vi "Read command in.vi"(8 "error in (no error)":errorcluster, 11 "Motor in":refnum<class "Motor.lvclass">) -> (0 "error out":errorcluster, 1 "action not empty":bool, 2 "command in":T1, 3 "Motor out":refnum<class "Motor.lvclass">)   [LabVIEW 2018, in "Motor.lvclass"]
uses:
  Motor.lvclass
  Motor.lvclass/Motor.ctl
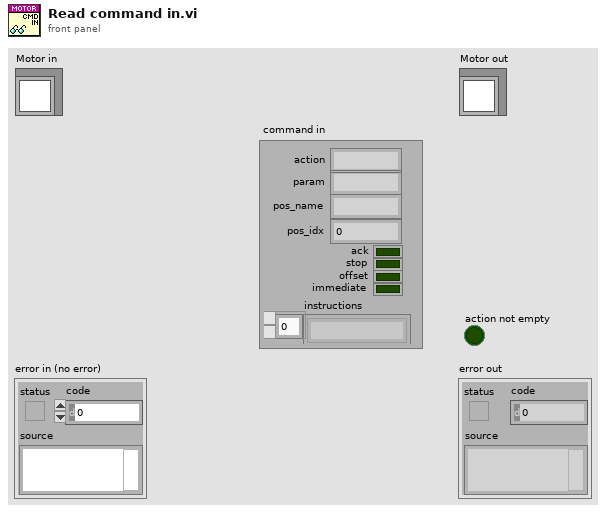
[diagram p1: front panel]
types:
  T1 = cluster{"action":string, "param":string, "pos_name":string, "pos_idx":i32, "ack":bool, "stop":bool, "offset":bool, "immediate":bool, "instructions":string[]}
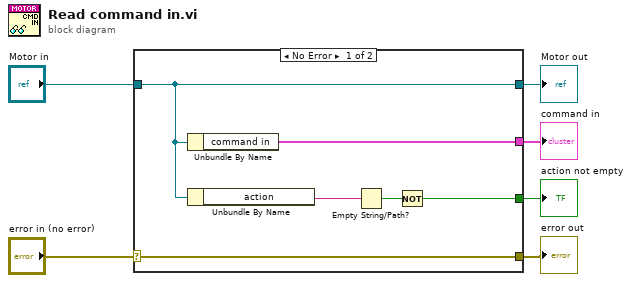
[diagram p0: block diagram]
diagram:
  n1 = case shown="No Error" "error in (no error)" {
    selector: "error in (no error)" -> [w12 w13]
    tunnel: [w12 w13] -> w5
    tunnel: [w10 w14] -> w3
    tunnel: "Motor in" -> [w10 w14]
    tunnel: [w11 _] -> w1
    tunnel: [w7 _] -> w2
    frame No Error {
      n2 = Unbundle By Name(w10) -> ("command in"=w11:T1)
      n3 = Unbundle By Name(w10) -> ("action"=w8:string)
      n4 = Empty String/Path?(string/path=w8) -> (empty?=w9:bool)
      n5 = Not(x=w9) -> (.not. x?=w7:bool)
    }
    frame Error {
    }
  }
  "error out" <- w5
  "Motor out" <- w3
  "action not empty" <- w2
  "command in" <- w1
